vi "Noise_measurement.vi"(0 "Gain (V/A)":dbl=100000000000.0, 1 "Cycles":i32, 3 "Lower Cut-Off":dbl=100.0, 5 "minimum value":dbl=-5.0 format="%0.2f", 7 "Filter On":bool, 9 "maximum value":dbl=5.0 format="%0.2f", 11 "physical channels":tag, 12 "rate":dbl=1000.0 format="%0.2f", 14 "samples per channel":i32=1000) -> (4 "Current (pA) Filtered":waveform(dbl)(graph), 6 "PSD (pA/Hz^1/2) Peaks Removed":cluster{"f0":dbl, "df":dbl, "magnitude":dbl[]}(graph), 10 "Current (pA)":dbl[](graph), 15 "PSD (pA/Hz^1/2)":cluster{"f0":dbl, "df":dbl, "magnitude":dbl[]}(graph))   [LabVIEW 2015]
uses:
  <vilib>/DAQmx/read.llb/DAQmx Read (Analog 1D DBL 1Chan NSamp).vi
  <vilib>/Analysis/baseanly.llb/Mean (DBL).vi
  <vilib>/DAQmx/create/channels.llb/DAQmx Create Channel (AI-Voltage-Basic).vi
  <vilib>/DAQmx/configure/timing.llb/DAQmx Timing (Sample Clock).vi
  <vilib>/DAQmx/miscellaneous.llb/DAQmx Fill In Error Info.vi
  <vilib>/express/express analysis/Spectral/Block/exnSpectralBlock spectral measurements PSD poly.vi
  <vilib>/express/express analysis/Spectral/Block/exnSpectralBlock spectral measurements PSD WFM.vi
  <vilib>/express/express analysis/Spectral/XNode/ExpressSpectralMeasurementsBlockNode.xnode
  <vilib>/Analysis/NI_AALBase.lvlib
panel:
  out "Current (pA) 2":dbl[](graph)
  in  "sample mode":i32(ring)=10178 items=["Finite Samples"=10178, "Continuous Samples"=10123, "Hardware Timed Single Point"=12522]
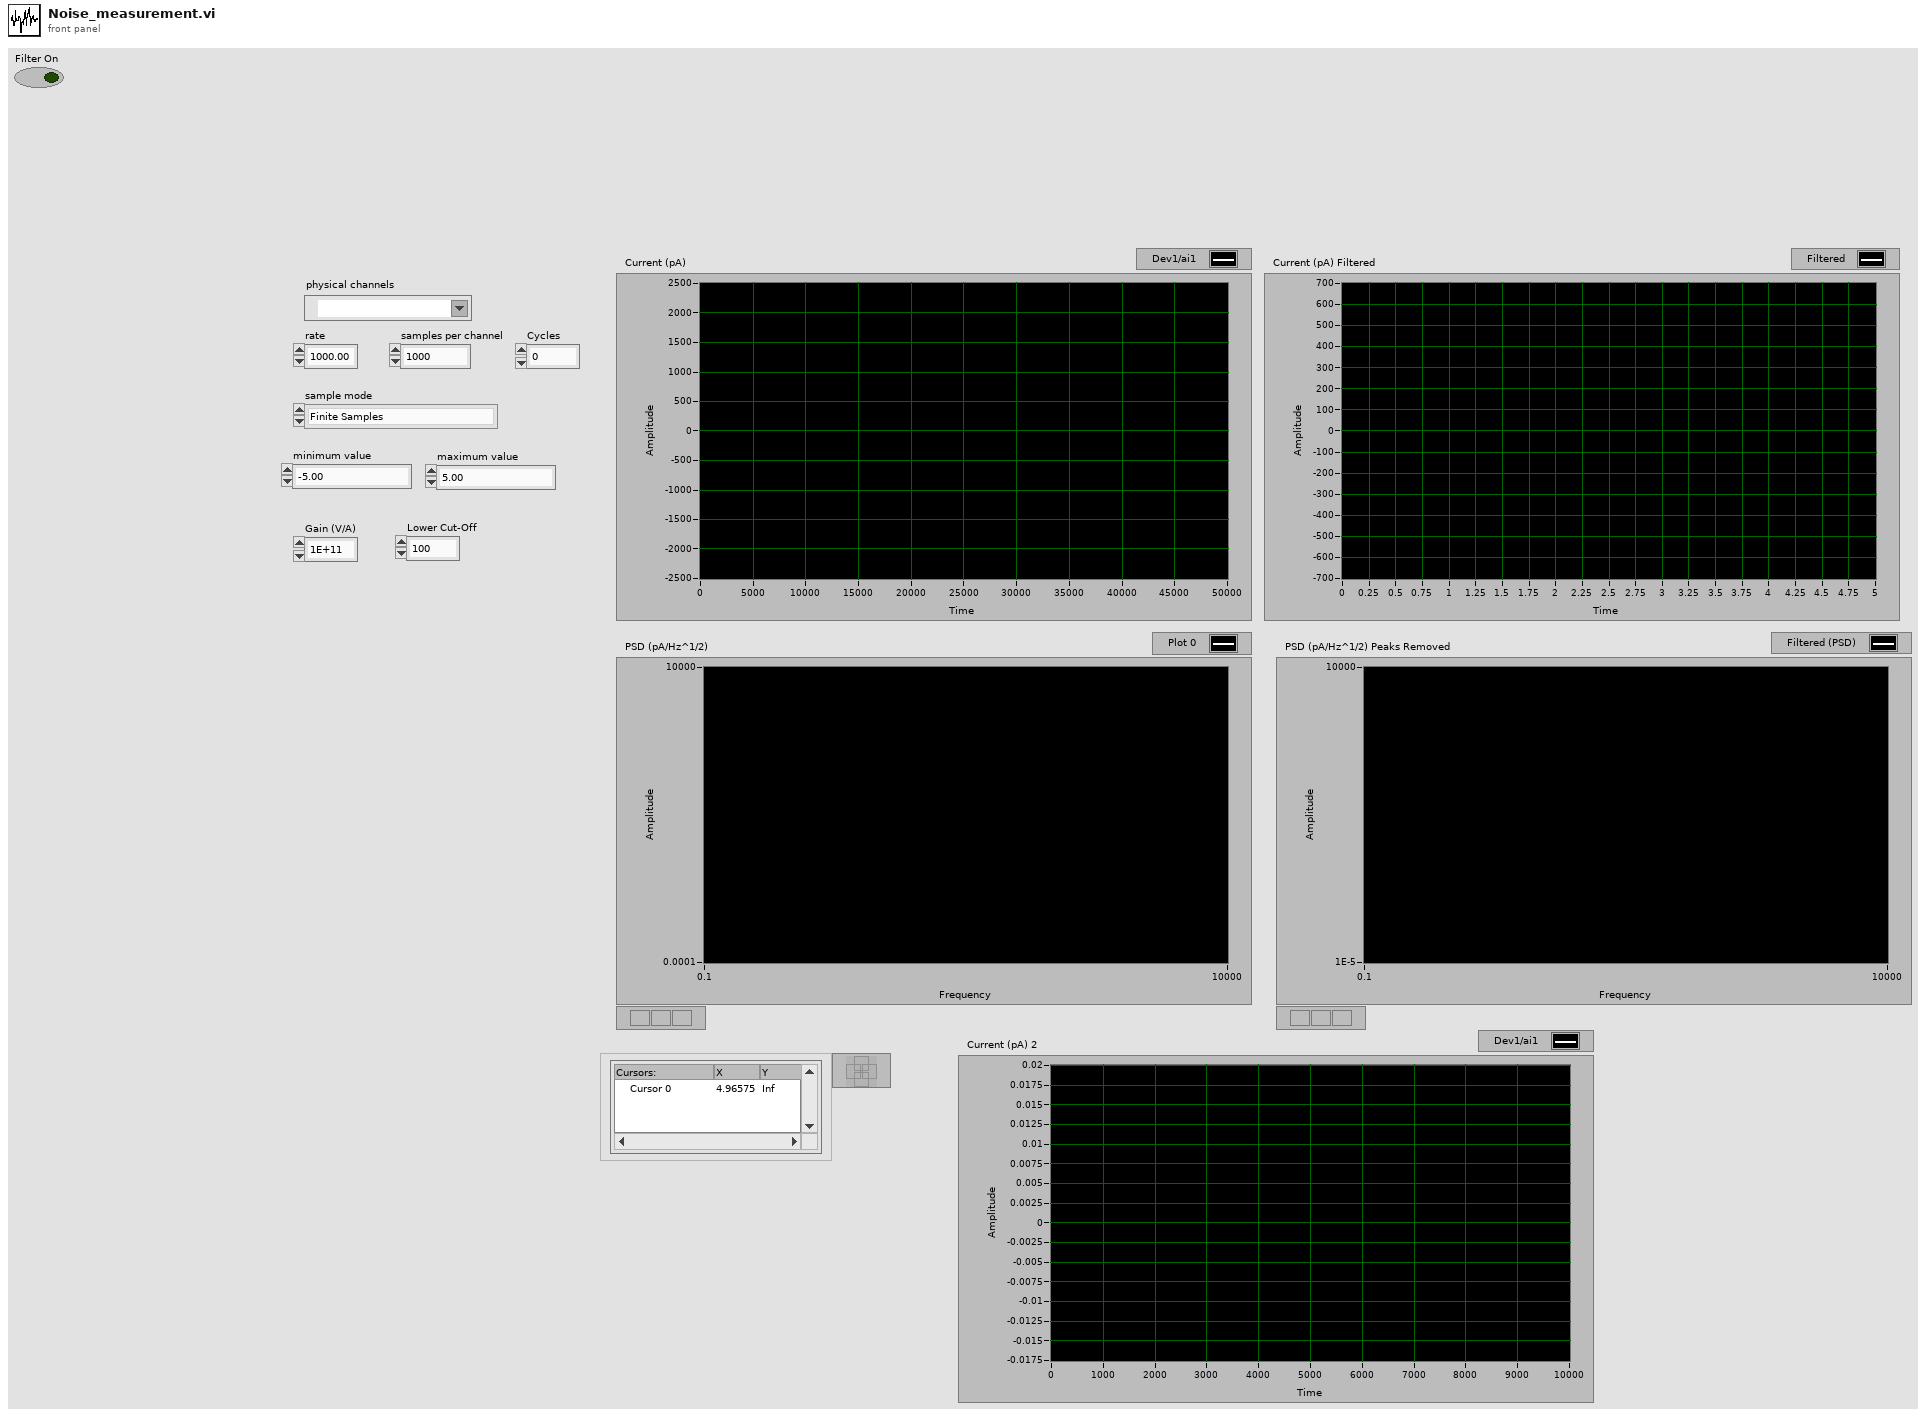
[diagram p1: front panel]
types:
  T1 = cluster{"averaging mode":u16, "weighting mode":u16, "number of averages":u32}
  T2 = cluster{"dB On (F)":bool, "unwrap phase (F)":bool, "convert to degree (F)":bool}
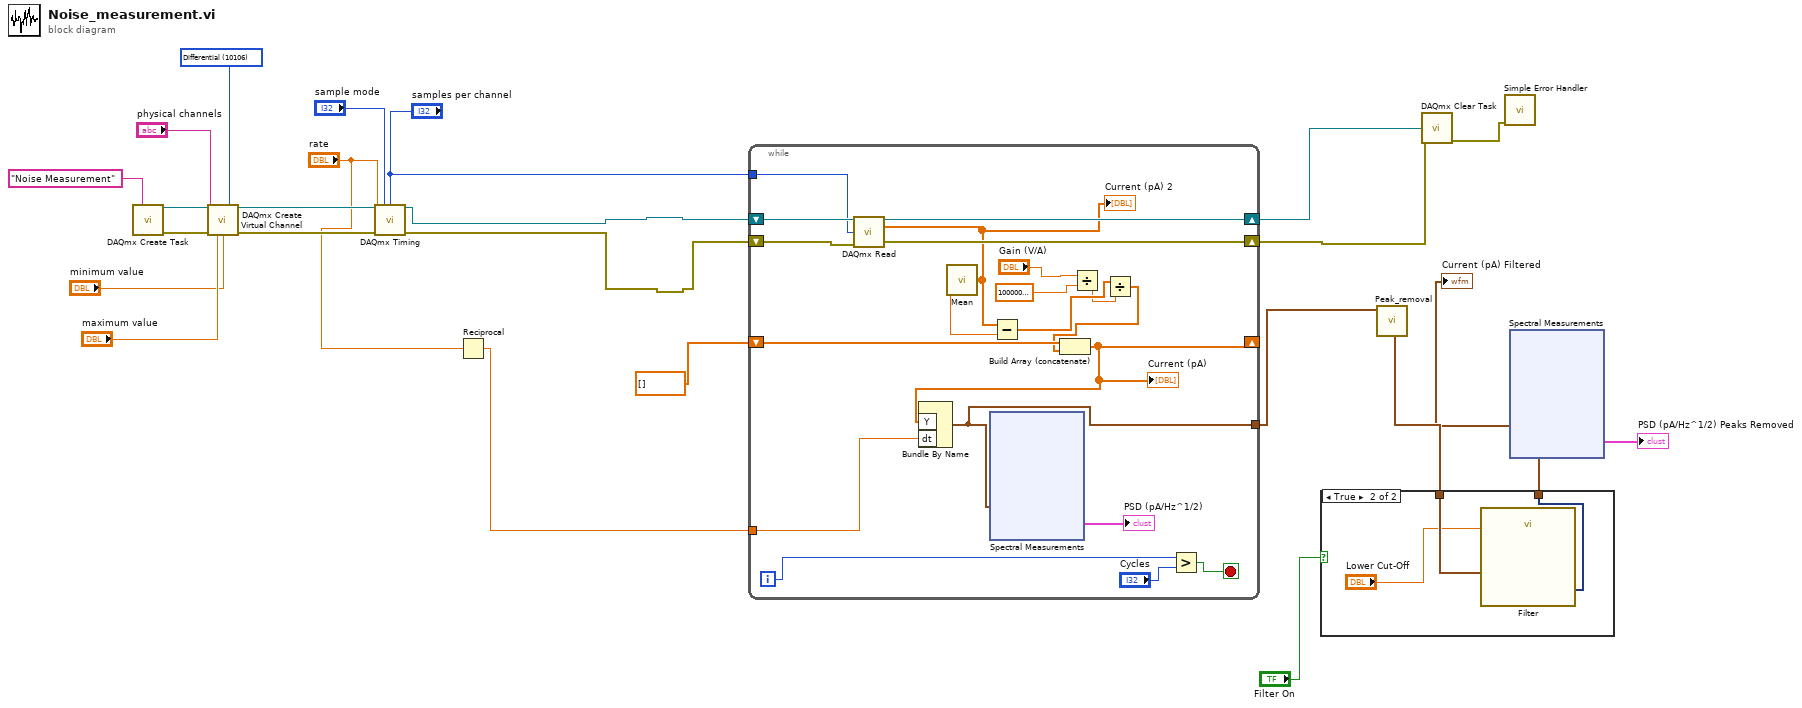
[diagram p0: block diagram]
diagram:
  w13 = 10106 items=["Default"=-1, "RSE"=10083, "NRSE"=10078, "Differential"=10106, "Pseudodifferential"=12529] ("input terminal configuration")
  n1 = call <vilib>:"DAQmx Create Task.vi"("new task name"="Noise Measurement") -> ("task out"=w22:refnum<k21>, "error out"=w24:errorcluster)  [unwired: 13 in]
  n2 = call-poly <vilib>:"DAQmx Create Virtual Channel.vi"("task in"=w22, "maximum value"="maximum value", "minimum value"="minimum value", "input terminal configuration"=w13, "physical channels"="physical channels", "error in"=w24) -> ("task out"=w21:refnum<k21>, "error out"=w23:errorcluster)  [unwired: 8 in]
  n3 = call-poly <vilib>:"DAQmx Timing.vi"("task/channels in"=w21, "sample mode"="sample mode", "samples per channel"="samples per channel", "rate"="rate", "error in"=w23) -> ("task out"=w2:refnum<k21>, "error out"=w1:errorcluster)  [unwired: 9 in]
  n4 = Reciprocal(x="rate") -> (1/x=w7:dbl)
  n5 = while {
    tunnel: "samples per channel" -> [w40]
    shift-right: [w42] -> w19
    shift-left: w1 -> [w44]
    shift-right: [w43] -> w20
    shift-left: w2 -> [w41]
    tunnel: w7 -> [w34]
    shift-right: [w37] -> _
    shift-left: dbl[] [] -> [w36]
    tunnel: [w35] -> w8
    i -> [w27]
    stop <- w26 stop-if-true
    n6 = call-poly <vilib>:"DAQmx Read.vi"("task/channels in"=w41, "number of samples per channel"=w40, "error in"=w44) -> ("task out"=w43:refnum<k21>, "data"=w30:dbl[], "error out"=w42:errorcluster)  [unwired: 10 in]
    "Current (pA) 2" <- w30
    n7 = call-poly <vilib>:"Mean.vi"("X"=w30) -> ("mean"=w39:dbl)  [unwired: 1 out]
    n8 = Subtract(x=w30, y=w39) -> (x-y=w29:dbl[])
    n9 = Divide(x="Gain (V/A)", y=1000000000000.0) -> (x/y=w28:dbl)
    n10 = Divide(x=w29, y=w28) -> (x/y=w31:dbl[])
    n11 = Build Array (concatenate)(w36, w31) -> (w37:dbl[])
    "Current (pA)" <- w37
    n12 = Bundle By Name("Y"=w37, "dt"=w34) -> (w35:waveform(dbl))  [unwired: 1 in]
    n13 = xnode "Spectral Measurements"("Signals"=w35) -> ("PSD"=→"PSD (pA/Hz^1/2)":cluster{"f0":dbl, "df":dbl, "magnitude":dbl[]})  [unwired: 1 in, 1 out]
    n14 = Greater?(x=w27, y="Cycles") -> (0:w26:bool)
  }
  n15 = call "Peak_removal.vi"("Input Waveform"=w8) -> ("Peaks Removed"=w5:waveform(dbl))  [unwired: 9 in, 1 out]
  n16 = case shown="True" "Filter On" {
    tunnel: w5 -> [w54 w57]
    tunnel: [w54 w56] -> w4
    frame False {
    }
    frame True {
      n17 = call "Filter"("Lower Cut-Off"="Lower Cut-Off", "Signal"=w57) -> ("Filtered Signal"=w56:dynamicdata)  [unwired: 8 in, 1 out]
    }
  }
  "Current (pA) Filtered" <- w4
  n18 = call <vilib>:"DAQmx Clear Task.vi"("task in"=w20, "error in"=w19) -> ("error out"=w18:errorcluster)  [unwired: 13 in]
  n19 = call <vilib>:"Simple Error Handler.vi"("error in (no error)"=w18) -> ()  [unwired: 4 in, 5 out]
  n20 = xnode "Spectral Measurements"("Signals"=w4) -> ("PSD"=→"PSD (pA/Hz^1/2) Peaks Removed":cluster{"f0":dbl, "df":dbl, "magnitude":dbl[]})  [unwired: 1 in, 1 out]
